vi "QI_radial profile normalization.vi"(11 "rp输入":dbl[](array[numeric])) -> (3 "rp输出":dbl[](array[numeric]))   [LabVIEW 2017]
uses:
  <vilib>/Analysis/5stat.llb/RMS (DBL).vi
  <vilib>/Analysis/NI_AALBase.lvlib
  <vilib>/Analysis/NI_AALPro.lvlib
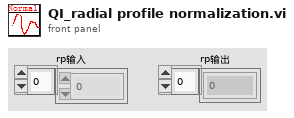
[diagram p1: front panel]
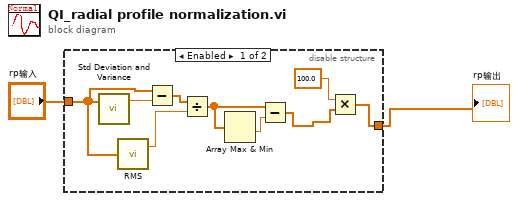
[diagram p0: block diagram]
diagram:
  n1 = disable-structure shown="Enabled" {
    disable-tunnel: "rp输入" -> [w9 w12]
    disable-tunnel: [w3 w12] -> w1
    frame Enabled {
      n2 = call <vilib>:"Std Deviation and Variance.vi"("X"=w9) -> ("mean"=w10:dbl)  [unwired: 1 in, 2 out]
      n3 = call-poly <vilib>:"RMS.vi"("X"=w9) -> ("rms value"=w8:dbl)  [unwired: 1 out]
      n4 = Subtract(x=w9, y=w10) -> (x-y=w11:dbl[])
      n5 = Divide(x=w11, y=w8) -> (x/y=w6:dbl[])
      n6 = Array Max & Min(array=w6) -> (min value=w7:dbl)  [unwired: 3 out]
      n7 = Subtract(x=w6, y=w7) -> (x-y=w4:dbl[])
      n8 = Multiply(x=100.0, y=w4) -> (x*y=w3:dbl[])
    }
    frame Disabled {
    }
  }
  "rp输出" <- w1
